vi "LineProtocol.vi"(8 "error in (no error)":errorcluster, 11 "DataPoint in":refnum<class "DataPoint.lvclass">) -> (0 "error out":errorcluster, 2 "Line protocol":string, 3 "DataPoint out":refnum<class "DataPoint.lvclass">)   [LabVIEW 2018, in "InfluxDB Client.lvlib" / "DataPoint.lvclass"]
uses:
  DataPoint.lvclass
  DataPoint.lvclass/DataPoint.ctl
  InfluxDB Client.lvlib
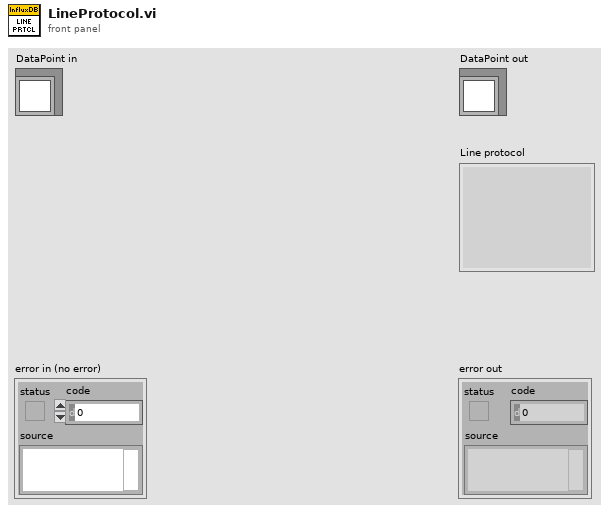
[diagram p1: front panel]
types:
  T1 = typedef "InfluxDB Client.lvlib/FieldSet.ctl" = cluster{"Key":string, "Value":variant}
  T2 = typedef "InfluxDB Client.lvlib/TagSet.ctl" = cluster{"Key":string, "Value":string}
  T3 = typedef "InfluxDB Client.lvlib/Precision.ctl" = enum16{"Seconds", "Milliseconds", "Nanoseconds"}
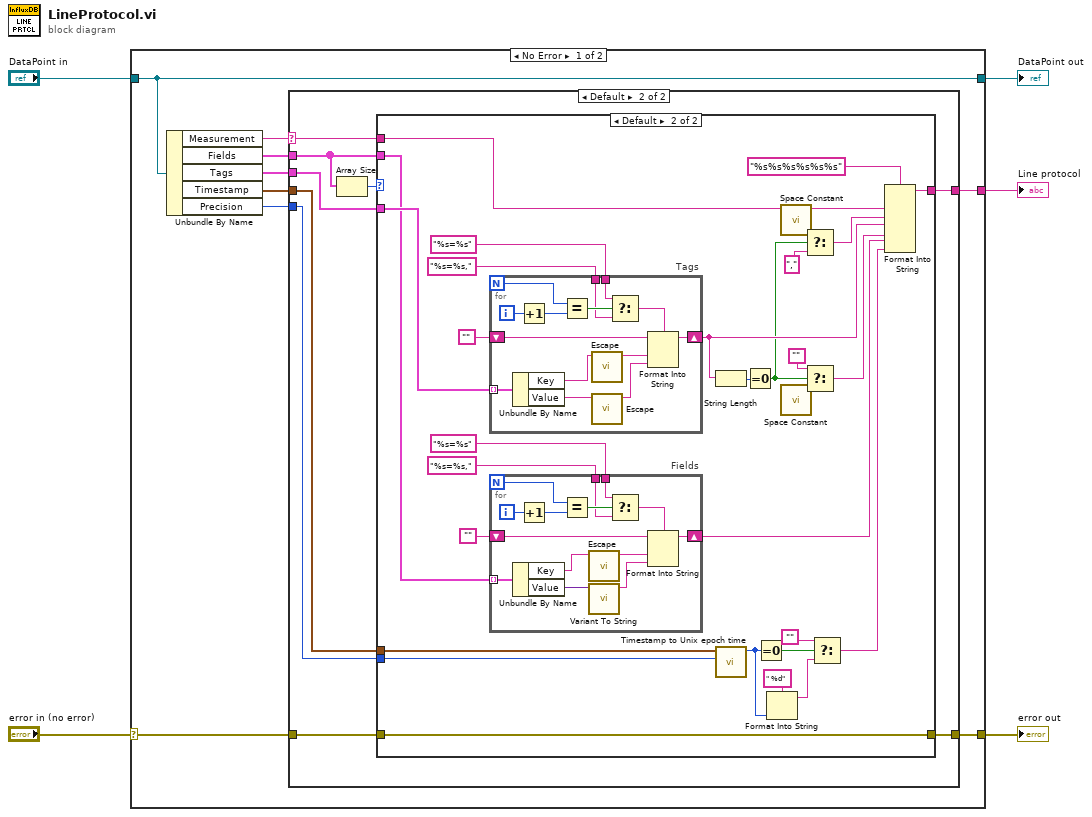
[diagram p0: block diagram]
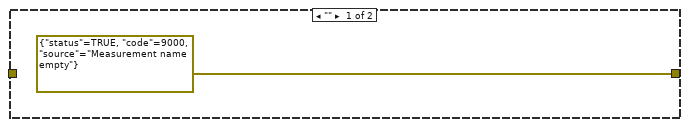
[diagram p2: hidden frame]
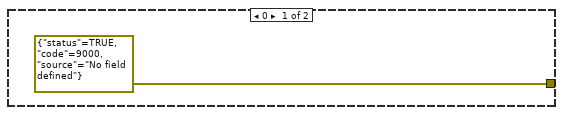
[diagram p3: hidden frame]
diagram:
  n1 = case shown="No Error" "error in (no error)" {
    selector: "error in (no error)" -> [w11 w85]
    tunnel: [w12 w85] -> w4
    tunnel: "DataPoint in" -> [w14 w84]
    tunnel: [w14 w84] -> w2
    tunnel: [w7 _] -> w1
    frame No Error {
      n2 = Unbundle By Name(w14) -> ("Measurement"=w13:string, "Fields"=w10:T1[], "Tags"=w9:T2[], "Timestamp"=w8:timestamp, "Precision"=w6:T3)
      n3 = case shown="Default" w13 {
        selector: w13 -> [_ w24]
        tunnel: [errorcluster {"status"=TRUE, "code"=9000, "source"="Measurement name empty"} ("error IO") w21] -> w12
        tunnel: w11 -> [_ w22]
        tunnel: w10 -> [_ w19]
        tunnel: w9 -> [_ w20]
        tunnel: w8 -> [_ w17]
        tunnel: [_ w18] -> w7
        tunnel: w6 -> [_ w16]
        frame "" {
        }
        frame Default {
          n4 = Array Size(array=w19) -> (size(s)=w23:i32)
          n5 = case shown="Default" w23 {
            tunnel: w24 -> [_ w53]
            tunnel: w22 -> [_ w55]
            tunnel: [errorcluster {"status"=TRUE, "code"=9000, "source"="No field defined"} ("error IO") w55] -> w21
            tunnel: w20 -> [_ w52]
            tunnel: w19 -> [_ w45]
            tunnel: [_ w43] -> w18
            tunnel: w17 -> [_ w42]
            tunnel: w16 -> [_ w26]
            frame 0 {
            }
            frame Default {
              n6 = for "Tags" {
                N -> [w81]
                tunnel: w52 -> [w74] mode=indexing
                shift-right: [w82] -> w34
                shift-left: "" -> [w83]
                tunnel: "%s=%s" ("format string") -> [w77]
                tunnel: "%s=%s," ("format string") -> [w76]
                i -> [w80]
                n7 = Unbundle By Name(w74) -> ("Key"=w73:string, "Value"=w71:string)
                n8 = Increment(x=w80) -> (x+1=w79:i32)
                n9 = Equal?(x=w81, y=w79) -> (x = y?=w78:bool)
                n10 = call "Escape.vi"("String in"=w73) -> ("String out"=w72:string)  [unwired: 10 in]
                n11 = call "Escape.vi"("String in"=w71) -> ("String out"=w70:string)  [unwired: 10 in]
                n12 = Select(t=w77, s=w78, f=w76) -> (s? t:f=w75:string)
                n13 = Format Into String(format string=w75, initial string=w83, w72, w70) -> (resulting string=w82:string)  [unwired: 1 in, 1 out]
              }
              n14 = for "Fields" {
                N -> [w67]
                tunnel: w45 -> [w60] mode=indexing
                shift-right: [w68] -> w35
                shift-left: "" -> [w69]
                tunnel: "%s=%s" ("format string") -> [w63]
                tunnel: "%s=%s," ("format string") -> [w62]
                i -> [w66]
                n15 = Unbundle By Name(w60) -> ("Key"=w57:string, "Value"=w59:variant)
                n16 = Increment(x=w66) -> (x+1=w65:i32)
                n17 = Equal?(x=w67, y=w65) -> (x = y?=w64:bool)
                n18 = call "Escape.vi"("String in"=w57) -> ("String out"=w56:string)  [unwired: 10 in]
                n19 = call "Variant To String.vi"("Variant"=w59) -> ("String"=w58:string)  [unwired: 9 in, 1 out]
                n20 = Select(t=w63, s=w64, f=w62) -> (s? t:f=w61:string)
                n21 = Format Into String(format string=w61, initial string=w69, w56, w58) -> (resulting string=w68:string)  [unwired: 1 in, 1 out]
              }
              n22 = String Length(string=w34) -> (length=w44:i32)
              n23 = call "Timestamp to Unix epoch time.vi"("Precision (ns)"=w26, "Timestamp"=w42) -> ("Unix epoch time"=w39:u64)  [unwired: 9 in]
              n24 = Equal To 0?(x=w44) -> (x = 0?=w28:bool)
              n25 = Equal To 0?(x=w39) -> (x = 0?=w41:bool)
              n26 = Format Into String(format string=" %d", w39) -> (resulting string=w37:string)  [unwired: 2 in, 1 out]
              n27 = call <vilib>:"Space Constant.vi"() -> ("String"=w33:string)
              n28 = call <vilib>:"Space Constant.vi"() -> ("String"=w30:string)
              n29 = Select(t=w33, s=w28, f="," ("input 2")) -> (s? t:f=w32:string)
              n30 = Select(t="" ("input 2"), s=w28, f=w30) -> (s? t:f=w27:string)
              n31 = Select(t="", s=w41, f=w37) -> (s? t:f=w36:string)
              n32 = Format Into String(format string="%s%s%s%s%s%s", w53, w32, w34, w27, w35, w36) -> (resulting string=w43:string)  [unwired: 2 in, 1 out]
            }
          }
        }
      }
    }
    frame Error {
    }
  }
  "error out" <- w4
  "DataPoint out" <- w2
  "Line protocol" <- w1
